vi "Session info dialog.vi"(8 "Error In":errorcluster, 11 "Session properties in":T1) -> (0 "Error Out":errorcluster, 3 "Session properties out":T1)   [LabVIEW 2019]
doc: "Displays information about a session"
uses:
  Type defs/Session properties Type Def.ctl
panel:
  in  "Cancel":bool
  in  "Apply":bool
  in  "Edit":bool
  out "myDLTS version":string
  out "Modified":string
  out "Created":string
  in  "Comment":string
  in  "Author":string
  in  "Session Name":string
  out "Type":enum16{"Text based", "Binary"}(ring) caption="Enum"
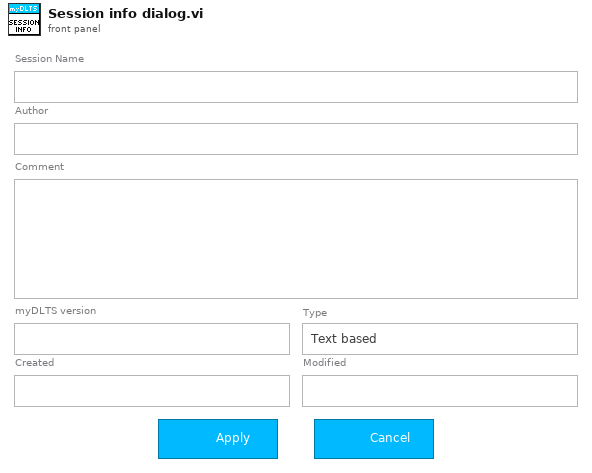
[diagram p1: front panel]
types:
  T1 = typedef "Session properties Type Def.ctl" = cluster{"Session name":string, "Comment":string, "User":string, "Software version":dbl, "Created":timestamp, "Modified":timestamp, "Binary":bool, "GUID":string}
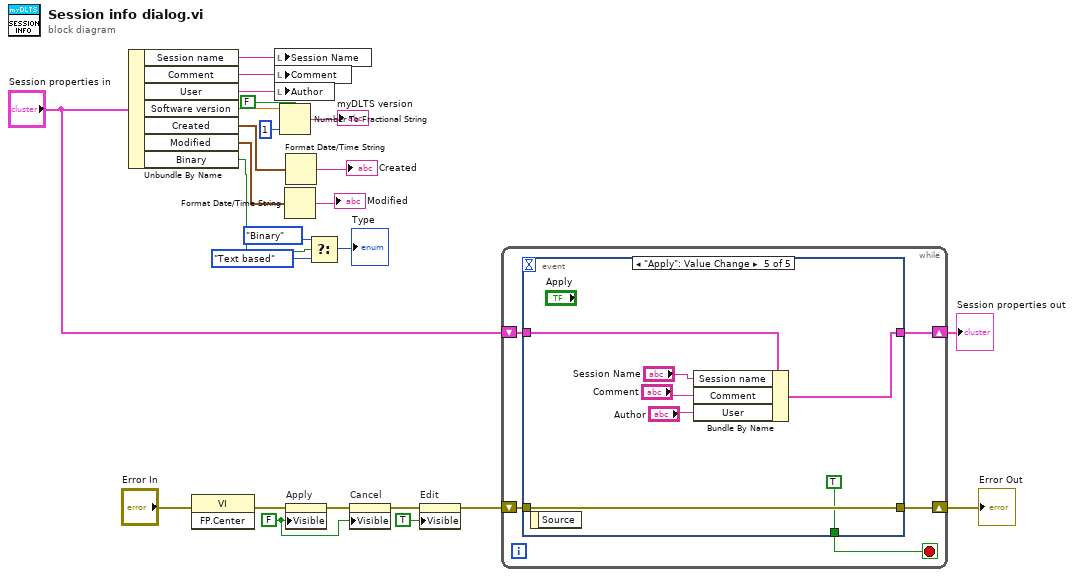
[diagram p0: block diagram]
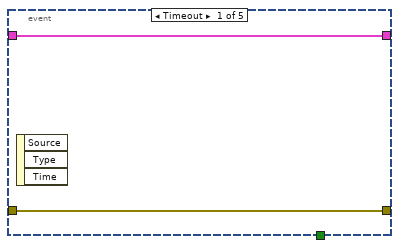
[diagram p2: hidden frame]
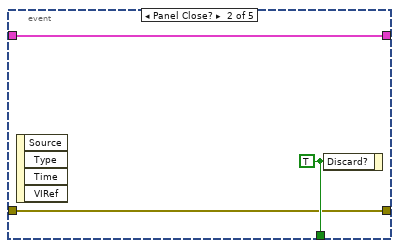
[diagram p3: hidden frame]
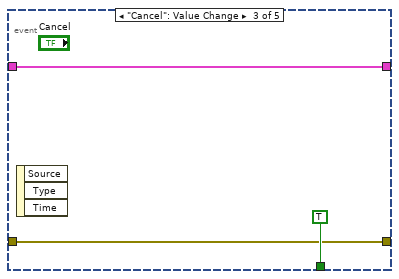
[diagram p4: hidden frame]
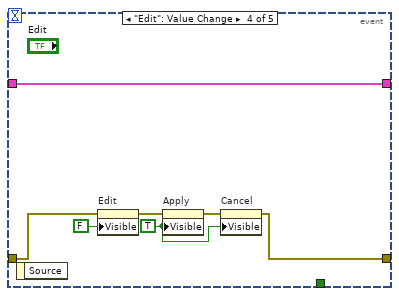
[diagram p5: hidden frame]
diagram:
  w11 = FALSE ("Visible")
  n1 = Unbundle By Name("Session properties in") -> ("Session name"=w10:string, "Comment"=w8:string, "User"=w9:string, "Software version"=w24:dbl, "Created"=w22:timestamp, "Modified"=w21:timestamp, "Binary"=w18:bool)
  n2 = invoke class="VI" method="FP.Center"(error in="Error In") -> (error out=w5:errorcluster)  [unwired: 2 in, 2 out]
  n3 = local write "Session Name"(w10) -> ()
  n4 = local write "Comment"(w8) -> ()
  n5 = local write "Author"(w9) -> ()
  n6 = Number To Fractional String(use system decimal point (T)=FALSE, number=w24, precision (6)=i16 1) -> (F-format string=→"myDLTS version":string)  [unwired: 1 in]
  n7 = Format Date/Time String(seconds (now)=w21) -> (date/time string=→"Modified":string)  [unwired: 2 in]
  n8 = Format Date/Time String(seconds (now)=w22) -> (date/time string=→"Created":string)  [unwired: 2 in]
  n9 = property on="Apply" class="Bool"(error in=w5, "Visible"=w11) -> (error out=w12:errorcluster)  [unwired: 1 in, 1 out]
  n10 = Select(t=enum16{"Text based", "Binary"}."Binary" ("Type"), s=w18, f=enum16{"Text based", "Binary"}."Text based") -> (s? t:f=→"Type":enum16{"Text based", "Binary"})
  n11 = property on="Cancel" class="Bool"(error in=w12, "Visible"=w11) -> (error out=w6:errorcluster)  [unwired: 1 in, 1 out]
  n12 = property on="Edit" class="Bool"(error in=w6, "Visible"=TRUE) -> (error out=w4:errorcluster)  [unwired: 1 in, 1 out]
  n13 = while {
    shift-right: [w27] -> w1
    shift-left: "Session properties in" -> [w28]
    shift-right: [w26] -> w2
    shift-left: w4 -> [w29]
    stop <- w30 stop-if-true
    n14 = event shown="[4] \"Apply\": Value Change" {
      selector: _ -> [_ _ _ _ _]
      dyn-events: _ -> [_ _ _ _ _]
      timeout: _ -> [_ _ _ _ _]
      tunnel: [_ w35 TRUE ("Discard?") _ TRUE ("Discard?")] -> w30
      tunnel: w29 -> [w31 w33 w36 w40 w47]
      tunnel: w28 -> [w32 w34 w38 w41 w52]
      tunnel: [w32 w34 w38 w41 w51] -> w27
      tunnel: [w31 w33 w36 w39 w47] -> w26
      event Timeout {
        n15 = event-data() -> ()  [unwired: 1 in, 3 out]
      }
      event Panel Close? {
        w35 = TRUE ("Discard?")
        n16 = event-data() -> ()  [unwired: 1 in, 4 out]
        n17 = event-data("Discard?"=w35) -> ()  [unwired: 1 in, 1 out]
      }
      event "Cancel": Value Change {
        n18 = event-data() -> ()  [unwired: 1 in, 3 out]
      }
      event "Edit": Value Change {
        w42 = TRUE ("Visible")
        n19 = event-data() -> ()  [unwired: 1 in, 1 out]
        n20 = property on="Edit" class="Bool"(error in=w40, "Visible"=FALSE) -> (error out=w44:errorcluster)  [unwired: 1 in, 1 out]
        n21 = property on="Apply" class="Bool"(error in=w44, "Visible"=w42) -> (error out=w43:errorcluster)  [unwired: 1 in, 1 out]
        n22 = property on="Cancel" class="Bool"(error in=w43, "Visible"=w42) -> (error out=w39:errorcluster)  [unwired: 1 in, 1 out]
      }
      event "Apply": Value Change {
        n23 = event-data() -> ()  [unwired: 1 in, 1 out]
        n24 = Bundle By Name(cluster=w52, "Session name"="Session Name", "Comment"="Comment", "User"="Author") -> (w51:T1)
      }
    }
  }
  "Error Out" <- w2
  "Session properties out" <- w1
